vi "speis.vi"(0 "IP adress":string="192.109.209.229", 1 "stop":bool, 2 "Channel":u8(ring)=4 items=["1", "2", "3", "4", "5", "6", "7", "8", "9", "10", "11", "12", "13", "14", "15", "16"], 3 "SPEIS Parameters":T2={"Step_number"=2, "Initial_Voltage_step"=0.0, "vs_initial"=TRUE, "Final_Voltage_step"=1.0, "vs_final"=FALSE, "Duration_step"=1.0, "Record_every_dI"=0.1, "Record_every_dT"=0.1, "Initial_frequency"=100000.0, "sweep"=FALSE, "Final_frequency"=1.0, "Frequency_number"=51, "Amplitude_Voltage"=0.01, "Wait_for_steady"=2.0, "Average_N_times"=1, "Correction"=TRUE, "I_Range"=12, "Bandwidth"=5, "em"=1, "ce"=0} {"ce" items=["Standard", "CE to ground"]; "Initial_Voltage_step" min=-10 max=10 format="%.5f"; "Step_number" min=0 step=1; "I_Range" items=["1pA", "1nA", "10nA", "100nA", "1µA", "10µA", "100µA", "1mA", "10mA", "100mA", "1A", "Booster", "Auto"]; "Wait_for_steady" min=0 format="%.2f"; "Record_every_dT" min=0 format="%.2e"; "Record_every_dI" min=0 format="%.2e"; "Duration_step" min=0 format="%.5f"; "Final_Voltage_step" min=-10 max=10 format="%.5f"; "Bandwidth" items=["1"=1, "2"=2, "3"=3, "4"=4, "5"=5, "6"=6, "7"=7, "8"=8, "9"=9]; "Average_N_times" min=1 max=1000 step=1; "Amplitude_Voltage" min=0.0005 max=0.5 format="%.2e"; "Final_frequency" min=1e-05 max=1000000 format="%.2e"; "Frequency_number" min=1 max=10000; "Initial_frequency" min=1e-05 max=1000000 format="%.2e"}, 4 "Exit":bool, 5 "Start":bool, 8 "Draw":T1(ring)) -> (6 "XY Graph":cluster{"Data p1":sgl[], "Data p1":dbl[]}[](graph)=[{"Data p1"=[525.50006, 538.618, 558.7457, 587.3537, 630.11804, 690.5473, 769.1625, 866.5284, 976.17816, 1089.6279, 1189.7482, 1279.7397, 1345.3214, 1394.7092, 1431.7653, 1455.0223, 1469.8767, 1479.4921, 1485.3942, 1488.4973, 1493.599, 1495.9125, 1499.4656, 1502.3853, 1506.3972, 1509.198, 1519.7369, 1532.5125, 1548.5372, 1580.3093, 1625.0144, 1694.3768, 1801.5819, 1957.731, 2171.8762, 2461.144, 2817.8232, 3216.9392, 3619.0576, 3986.1555, 4300.8384, 4536.2026, 4707.0835, 4828.639, 4904.999, 4961.0366, 4994.4067, 5015.1143, 5029.5254, 5037.418, 5042.429, 525.3447, 538.11237, 558.4203, 587.67224, 630.1018, 689.9828, 768.2711, 865.9559, 975.45575, 1088.0951, 1190.5238, 1279.0249, 1347.1433, 1396.1802, 1430.4937, 1455.2814, 1469.1127, 1480.9547, 1488.2792, 1491.4941, 1493.8552, 1496.4435, 1497.5511, 1502.2585, 1506.1387, 1509.9863, 1518.135, 1530.0344, 1549.0596, 1579.7124, 1625.0818, 1698.2051, 1802.8951, 1952.263, 2172.5627, 2465.0474, 2821.2722, 3224.1062, 3621.5154, 4006.4937, 4287.0464, 4530.4033, 4711.4463, 4846.2896, 4918.22, 4963.792, 5006.571, 5024.125, 5036.2017, 5047.449, 5051.315, 525.54193, 538.3897, 557.91473, 588.05676, 630.4936, 689.3102, 769.6545, 866.44385, 976.8946, 1088.5287, 1191.8607, 1279.7543, 1347.9636, 1396.8135, 1430.9287, 1453.9589, 1470.3905, 1480.8995, 1486.5005, 1491.8065, 1494.8728, 1495.035, 1497.364, 1502.3115, 1506.6406, 1509.7494, 1520.2966, 1532.3849, 1551.5309, 1581.3643, 1626.9884, 1696.2556, 1800.7041, 1954.6533, 2176.5808, 2462.342, 2819.6333, 3220.7124, 3630.4177, 3998.0688, 4306.804, 4559.2373, 4719.661, 4837.343, 4913.759, 4967.9824, 5011.7876, 5025.0054, 5040.9824, 5049.399, 5058.189], "Data p1"=[-150.71189880371094, -185.61993408203125, -228.1602783203125, -277.7409362792969, -332.0828552246094, -388.3536071777344, -440.2685852050781, -479.6073303222656, -497.4354248046875, -492.5791931152344, -463.5277404785156, -416.0335998535156, -364.6885070800781, -311.1602783203125, -263.2023010253906, -222.48780822753906, -189.07347106933594, -164.32290649414062, -147.07318115234375, -137.23709106445312, -134.4752197265625, -138.10047912597656, -152.14559936523438, -170.2203369140625, -199.28997802734375, -238.3840789794922, -290.4477233886719, -355.0041809082031, -435.4027404785156, -539.1777954101562, -667.4210815429688, -821.8733520507812, -997.7675170898438, -1197.373291015625, -1394.82568359375, -1582.048095703125, -1717.46923828125, -1778.4962158203125, -1742.513427734375, -1633.1392822265625, -1453.841064453125, -1255.0560302734375, -1052.457275390625, -865.8721923828125, -707.827880859375, -570.5523681640625, -455.1785888671875, -364.49017333984375, -289.9132995605469, -231.135009765625, -183.6439971923828, -150.6773681640625, -185.84783935546875, -228.77284240722656, -278.3961181640625, -332.7877502441406, -388.551513671875, -440.7836608886719, -479.08306884765625, -499.46099853515625, -492.4226989746094, -464.9497985839844, -416.5841979980469, -364.1741027832031, -310.4356994628906, -262.843017578125, -223.28204345703125, -189.56234741210938, -164.49154663085938, -148.58004760742188, -137.69810485839844, -135.09109497070312, -138.912841796875, -151.2158966064453, -170.32308959960938, -196.95445251464844, -236.5548095703125, -289.3612976074219, -354.9062194824219, -435.35992431640625, -540.9880981445312, -668.5939331054688, -821.7505493164062, -993.9796752929688, -1198.608154296875, -1398.090087890625, -1581.3919677734375, -1721.475341796875, -1777.119140625, -1735.2742919921875, -1629.3763427734375, -1462.967529296875, -1237.9119873046875, -1051.7672119140625, -870.1654663085938, -707.5675048828125, -580.3982543945312, -455.0499572753906, -364.8717041015625, -287.6647033691406, -226.23031616210938, -186.34091186523438, -150.48431396484375, -185.98463439941406, -228.33602905273438, -277.496337890625, -332.2249450683594, -388.3759460449219, -440.437255859375, -480.6752624511719, -497.97943115234375, -490.92437744140625, -463.6277160644531, -416.9968566894531, -364.2229309082031, -311.0670471191406, -263.4906311035156, -221.8280487060547, -190.08363342285156, -165.50880432128906, -145.69888305664062, -135.96371459960938, -134.3701934814453, -139.62152099609375, -151.39317321777344, -170.60525512695312, -198.75314331054688, -237.4167022705078, -288.7137756347656, -355.7140808105469, -437.6841735839844, -539.8258666992188, -668.255859375, -819.745361328125, -995.9793701171875, -1194.9197998046875, -1398.14892578125, -1591.957763671875, -1718.02490234375, -1787.792236328125, -1749.94580078125, -1622.7584228515625, -1456.0980224609375, -1251.5211181640625, -1044.2322998046875, -868.7525024414062, -706.819580078125, -570.400390625, -455.4763488769531, -364.127197265625, -294.8734130859375, -231.19313049316406, -184.1147003173828]}], 7 "Number of points":i32=153)   [LabVIEW 2012]
doc: "The Staircase Potentio Electrochemical Impedance Spectroscopy (SPEIS) technique is designed to perform successive impedance measurements (on a whole frequency range) during a potential sweep. \nThis technique consists in a staircase potential sweep (potential limits and number of steps defined by the user). An impedance measurement (with an adjustable number of frequencies) is performed on each potential step.\n\nIn general, in this VI, the first thing to do is to start by establishing the connection with the instrument defined by its IP adress, then load the firmware in the channel selected, get the information on the plugged channels, load protocol on a channel, start/stop the protocol, retreive data and draw the graph.\nThis technique is applied just for channels with impedance capabilities (Zboard)."
uses:
  base_xml.llb/Type Descriptor Enumeration__ogtk.ctl
panel:
  out "Data p0":sgl[][](array[numeric])=[[0.100008, 0.0009844337, 1.788816e-07, 1.0], [0.200016, 0.0010607007, 1.7521837e-07, 1.0], [0.300024, 0.0009844337, 1.7453168e-07, 1.0], [0.400032, 0.0009844337, 1.7399759e-07, 1.0], [0.50004, 0.0010607007, 1.7369238e-07, 1.0], [0.600048, 0.0007556325, 1.7285309e-07, 1.0], [0.700056, 0.0010607007, 1.7415019e-07, 1.0], [0.800064, 0.0009844337, 1.732346e-07, 1.0], [0.90007204, 0.00090816664, 1.729294e-07, 1.0], [31.67708, 0.5012512, 9.935654e-05, 1.0000001], [31.777088, 0.5012512, 9.9204015e-05, 1.0000001], [31.877096, 0.50132746, 9.912774e-05, 1.0000001], [31.977104, 0.50148, 9.935654e-05, 1.0000001], [32.07711, 0.5012512, 9.9204015e-05, 1.0000001], [32.17712, 0.5012512, 9.9204015e-05, 1.0000001], [32.277126, 0.5012512, 9.912774e-05, 1.0000001], [32.377136, 0.50132746, 9.9204015e-05, 1.0000001], [32.477142, 0.5011749, 9.912774e-05, 1.0000001], [60.111145, 0.96091276, 0.000400375, 1.0000002], [60.21115, 1.0013343, 0.00019804362, 1.0000002], [60.31116, 1.001258, 0.00019819614, 1.0000002], [60.411167, 1.0013343, 0.0001982724, 1.0000002], [60.511177, 1.0013343, 0.00019819614, 1.0000002], [60.611183, 1.0015631, 0.00019811987, 1.0000002], [60.711193, 1.001258, 0.00019819614, 1.0000002], [60.8112, 1.0013343, 0.0001982724, 1.0000002], [60.91121, 1.001258, 0.00019796735, 1.0000002], [61.011215, 1.001258, 0.00019804362, 1.0000002]]
  out "Data p1":sgl[][](array[numeric])=[[100031.24, 0.009869354, 1.8053093e-05, -0.27930045, 0.001764305, 3.9379972e-07, 0.0, 0.018222777, 1.8088715e-05, -0.025958419, -0.00018480215, -3.9379972e-07, 2.0, 2.029, 8.0, 1.0], [79437.5, 0.010228618, 1.7954228e-05, -0.33187628, 0.0017653664, 3.8618438e-07, 0.0, 0.01806867, 1.7994063e-05, -0.018080682, -0.00019200613, -3.861844e-07, 2.0, 2.114, 8.0, 1.0], [63093.75, 0.010669165, 1.7677803e-05, -0.3876784, 0.0017698539, 3.946376e-07, 0.0, 0.017742673, 1.7717768e-05, -0.015037537, -0.00018748268, -3.946376e-07, 2.0, 2.199, 8.0, 1.0], [50125.0, 0.0101253055, 1.5584323e-05, -0.44170764, 0.0017671726, 3.9245887e-07, 0.0, 0.015633836, 1.5619022e-05, -0.011037588, -0.00018580719, -3.924589e-07, 2.0, 2.368, 8.0, 1.0], [39812.496, 0.010687894, 1.5005408e-05, -0.48502678, 0.0017727586, 3.9467452e-07, 0.0, 0.015032693, 1.5036869e-05, -0.009105086, -0.00020297953, -3.9467454e-07, 2.0, 2.453, 8.0, 1.0], [31625.002, 0.010131325, 1.27878975e-05, -0.5123023, 0.0017680849, 3.9675982e-07, 0.0, 0.012788134, 1.2812633e-05, -0.005294323, -0.00019100076, -3.9675984e-07, 2.0, 2.622, 8.0, 1.0], [25124.996, 0.010685012, 1.2056367e-05, -0.51987815, 0.0017704311, 3.8622122e-07, 0.0, 0.012053828, 1.2077107e-05, -0.0034683943, -0.00018999552, -3.8622125e-07, 2.0, 2.707, 8.0, 1.0], [19953.123, 0.010150351, 1.0248726e-05, -0.5055121, 0.001768178, 3.9500952e-07, 0.0, 0.010238029, 1.0263841e-05, -0.0036523342, -0.00019217345, -3.9500955e-07, 2.0, 2.876, 8.0, 1.0], [15842.013, 0.010598964, 9.674011e-06, -0.4712778, 0.0017736709, 3.9139732e-07, 0.0, 0.009650077, 9.6858e-06, -0.0015640259, -0.00019803717, -3.9139735e-07, 2.0, 2.961, 8.0, 1.0], [12590.899, 0.010097275, 8.443992e-06, -0.42456722, 0.0017629458, 3.7616655e-07, 0.0, 0.008435441, 8.452159e-06, 2.670288e-05, -0.00016000666, -3.7616658e-07, 2.0, 3.161, 8.0, 1.0], [10019.525, 0.0104980795, 8.221826e-06, -0.3715102, 0.0017539338, 3.6335635e-07, 0.0, 0.008224506, 8.227834e-06, -0.00051116943, -0.0001420804, -3.633564e-07, 2.0, 3.28, 8.0, 1.0], [7944.256, 0.010987763, 8.165296e-06, -0.31431544, 0.0017541572, 3.568768e-07, 0.0, 0.0081453305, 8.16958e-06, -0.0020017624, -0.00012088722, -3.5687682e-07, 2.0, 3.425, 8.0, 1.0], [6322.935, 0.010157951, 7.287563e-06, -0.26471734, 0.0017405088, 3.52557e-07, 0.0, 0.0072648395, 7.2902762e-06, 0.0013228655, -0.00012222746, -3.5255704e-07, 2.0, 3.778, 8.0, 1.0], [5013.0186, 0.01075666, 7.5274156e-06, -0.21950568, 0.0017390565, 3.5142125e-07, 0.0, 0.00750066, 7.529323e-06, -0.0017416477, -0.0001242379, -3.5142128e-07, 2.0, 3.992, 8.0, 1.0], [3981.1804, 0.010172644, 6.987874e-06, -0.18180084, 0.0017367104, 3.4957787e-07, 0.0, 0.0069908933, 6.9890734e-06, -0.0010359287, -0.00012180861, -3.4957793e-07, 2.0, 4.42, 8.0, 1.0], [3160.0593, 0.010855657, 7.3750953e-06, -0.15173492, 0.0017394476, 3.489076e-07, 0.0, 0.007377897, 7.375971e-06, -0.00044322014, -0.00012591323, -3.4890766e-07, 2.0, 4.6349998, 8.0, 1.0], [2514.0195, 0.010156401, 6.853231e-06, -0.12792969, 0.0017408812, 3.498758e-07, 0.0, 0.006835944, 6.8537975e-06, 0.0020416975, -0.00014182905, -3.4987585e-07, 2.0, 5.062, 8.0, 1.0], [1993.0898, 0.010699353, 7.1875784e-06, -0.11061376, 0.001741235, 3.443086e-07, 0.0, 0.007164294, 7.1879995e-06, -0.0009522438, -0.00013546273, -3.4430863e-07, 2.0, 5.277, 8.0, 1.0], [1583.4792, 0.010107939, 6.771774e-06, -0.098691225, 0.0017376042, 3.4693392e-07, 0.0, 0.006733144, 6.7720653e-06, -0.0009715855, -0.00013630038, -3.4693397e-07, 2.0, 5.708, 8.0, 1.0], [1258.7904, 0.010411834, 6.965321e-06, -0.091938496, 0.001736487, 3.3749387e-07, 0.0, 0.0069400347, 6.965549e-06, -0.0020059347, -0.00013872965, -3.3749393e-07, 2.0, 5.9240003, 8.0, 1.0], [999.0409, 0.010659541, 7.108064e-06, -0.08979225, 0.0017378834, 3.385552e-07, 0.0, 0.0071048443, 7.108256e-06, -3.9339066e-06, -0.00013093927, -3.3855522e-07, 2.0, 6.1410003, 8.0, 1.0], [794.2393, 0.010820501, 7.2027497e-06, -0.092057616, 0.0017324092, 3.4103158e-07, 0.0, 0.007164113, 7.2029206e-06, 0.0011003017, -0.000125997, -3.4103164e-07, 2.0, 6.3580003, 8.0, 1.0], [631.00977, 0.010931326, 7.2529074e-06, -0.10112047, 0.0017288156, 3.4155292e-07, 0.0, 0.0072435015, 7.2530606e-06, 0.0020492077, -0.0001239028, -3.4155298e-07, 2.0, 6.576, 8.0, 1.0], [500.80118, 0.010105555, 6.683579e-06, -0.11281896, 0.001734774, 3.4153427e-07, 0.0, 0.006647158, 6.683726e-06, -0.0010091066, -0.00013177695, -3.4153433e-07, 2.0, 7.0090003, 8.0, 1.0], [398.5971, 0.010142034, 6.674487e-06, -0.13153195, 0.0017367849, 3.433962e-07, 0.0, 0.006641871, 6.6746197e-06, 0.0012131929, -0.00015238376, -3.4339627e-07, 2.0, 7.229, 8.0, 1.0], [316.3159, 0.0101667335, 6.654018e-06, -0.15665984, 0.0017379579, 3.4335898e-07, 0.0, 0.0066457815, 6.654146e-06, -0.001480341, -0.00015380779, -3.4335903e-07, 2.0, 7.448, 8.0, 1.0], [251.04433, 0.01018918, 6.585379e-06, -0.18883991, 0.0017377159, 3.436569e-07, 0.0, 0.0065762023, 6.5854924e-06, 0.002457559, -0.00014300179, -3.4365695e-07, 2.0, 7.669, 8.0, 1.0], [199.29855, 0.010201627, 6.4850747e-06, -0.22763349, 0.001744326, 3.450161e-07, 0.0, 0.0064792074, 6.485203e-06, -0.0012426376, -0.00014953566, -3.4501616e-07, 2.0, 7.895, 8.0, 1.0], [158.62956, 0.01019249, 6.3363113e-06, -0.27409363, 0.0017508802, 3.4900066e-07, 0.0, 0.0063282293, 6.336429e-06, -0.00015228987, -0.00014551482, -3.4900071e-07, 2.0, 8.123, 8.0, 1.0], [125.84552, 0.010199593, 6.108428e-06, -0.32880032, 0.0017499119, 3.396537e-07, 0.0, 0.006088465, 6.10855e-06, -0.0021110773, -0.00014844669, -3.3965375e-07, 2.0, 8.351, 8.0, 1.0], [99.90408, 0.010190543, 5.8008377e-06, -0.3897109, 0.0017508056, 3.446437e-07, 0.0, 0.005801017, 5.8009496e-06, 0.0016998751, -0.00014727394, -3.4464375e-07, 2.0, 8.585, 8.0, 1.0], [79.51632, 0.010190832, 5.4114853e-06, -0.4516238, 0.0017413839, 3.3969093e-07, 0.0, 0.005403216, 5.4116135e-06, -0.0005774498, -0.00014107513, -3.3969098e-07, 2.0, 8.826, 8.0, 1.0], [63.160732, 0.0101588145, 4.932837e-06, -0.50577784, 0.0017380696, 3.232843e-07, 0.0, 0.0048995684, 4.933435e-06, -0.0022892952, -0.00015162982, -3.2328435e-07, 2.0, 9.331, 7.0, 1.0], [50.08012, 0.0101338, 4.4158555e-06, -0.5489146, 0.0017423521, 3.2462907e-07, 0.0, 0.0044069523, 4.416364e-06, -0.0016965866, -0.00016863461, -3.2462918e-07, 2.0, 9.584, 7.0, 1.0], [39.85971, 0.010110853, 3.917116e-06, -0.57088757, 0.0017390565, 3.232749e-07, 0.0, 0.003909233, 3.917622e-06, 0.0017719865, -0.0001569909, -3.23275e-07, 2.0, 9.849, 7.0, 1.0], [31.58696, 0.010090547, 3.4488567e-06, -0.5713042, 0.001736487, 3.2309606e-07, 0.0, 0.0034521155, 3.4493996e-06, -0.003828764, -0.00017081253, -3.2309612e-07, 2.0, 10.116, 7.0, 1.0], [25.104433, 0.010081783, 3.05511e-06, -0.5473771, 0.0017249426, 3.2149413e-07, 0.0, 0.0030513897, 3.0555955e-06, 0.0057106614, -0.00014534722, -3.2149427e-07, 2.0, 10.409, 7.0, 1.0], [19.929855, 0.010076249, 2.7412152e-06, -0.5050314, 0.0017313849, 3.2125197e-07, 0.0, 0.0027353163, 2.7417095e-06, -0.0069835186, -0.00015146224, -3.212521e-07, 2.0, 10.725, 7.0, 1.0], [15.836134, 0.010059833, 2.5044978e-06, -0.44872427, 0.0017287785, 3.204436e-07, 0.0, 0.0025177128, 2.5049212e-06, 0.009344101, -0.00014677126, -3.2044363e-07, 2.0, 11.055, 7.0, 1.0], [12.600794, 0.010063741, 2.3362027e-06, -0.38884282, 0.0017246262, 3.186163e-07, 0.0, 0.0023388118, 2.3364873e-06, 0.0006400645, -0.00014635241, -3.186164e-07, 2.0, 11.465, 7.0, 1.0], [9.990409, 0.010058779, 2.2156298e-06, -0.32597756, 0.0017271581, 3.216877e-07, 0.0, 0.0022162707, 2.2159718e-06, -0.0044992566, -0.00015028955, -3.21688e-07, 2.0, 11.879, 7.0, 1.0], [7.939562, 0.010051124, 2.1355277e-06, -0.2699232, 0.0017190769, 3.1830135e-07, 0.0, 0.0021537226, 2.1358414e-06, -0.0010365248, -0.00014350438, -3.1830172e-07, 2.0, 12.397, 7.0, 1.0], [6.3004045, 0.010050946, 2.0838283e-06, -0.21997207, 0.0017442836, 3.3078075e-07, 0.0, 0.0020929575, 2.084185e-06, 0.00019574165, -0.00018570227, -3.307811e-07, 2.0, 13.045, 7.0, 1.0], [5.008012, 0.010055232, 2.049721e-06, -0.17743433, 0.001757515, 3.327263e-07, 0.0, 0.002057552, 2.0499922e-06, -0.0017228127, -0.00021201238, -3.3272647e-07, 2.0, 13.857, 7.0, 1.0], [3.9859712, 0.010047529, 2.027425e-06, -0.14331807, 0.0017548279, 3.3264936e-07, 0.0, 0.0020328981, 2.0277243e-06, -0.0021646023, -0.00020486997, -3.326495e-07, 2.0, 14.873, 7.0, 1.0], [3.1680837, 0.010054357, 2.0133932e-06, -0.11450362, 0.0017575176, 3.332066e-07, 0.0, 0.0020133706, 2.0137181e-06, 0.0010950565, -0.00020909487, -3.3320666e-07, 2.0, 16.148, 7.0, 1.0], [2.504006, 0.010050174, 2.0039806e-06, -0.09088659, 0.0017548916, 3.3225882e-07, 0.0, 0.002016635, 2.0043522e-06, -0.00028324127, -0.00023046214, -3.3225888e-07, 2.0, 17.759, 7.0, 1.0], [1.9879117, 0.010061348, 2.0009275e-06, -0.07255077, 0.0017483011, 3.1155264e-07, 0.0, 0.0020140824, 2.0043926e-06, -0.003084302, -0.00021901223, -3.1155272e-07, 2.0, 21.81, 6.0, 1.0], [1.5814751, 0.010062281, 1.9973268e-06, -0.057578564, 0.0017498633, 3.115516e-07, 0.0, 0.002005952, 2.0001908e-06, -0.0011792183, -0.00022941067, -3.1155167e-07, 2.0, 24.351, 6.0, 1.0], [1.2617111, 0.010061398, 1.9952333e-06, -0.04585147, 0.0017614333, 3.124857e-07, 0.0, 0.002001588, 1.9988286e-06, -0.00019466877, -0.00024342869, -3.124858e-07, 2.0, 27.535, 6.0, 1.0], [1.0000616, 0.010060886, 1.993924e-06, -0.036403656, 0.0017541798, 3.1092628e-07, 0.0, 0.0020091715, 1.9974327e-06, 0.0009430647, -0.00025171688, -3.109264e-07, 2.0, 31.547, 6.0, 1.0], [100031.24, 0.0098445695, 1.8012992e-05, -0.2793181, 0.5023526, 9.9444e-05, 0.0, 0.018171087, 1.8048326e-05, -0.026801586, -0.09870481, -9.9444056e-05, 2.0, 32.842, 8.0, 1.0000001], [79437.5, 0.010201275, 1.7918928e-05, -0.3325441, 0.5023489, 9.944558e-05, 0.0, 0.018042367, 1.7958415e-05, -0.019655943, -0.09869501, -9.944564e-05, 2.0, 32.927, 8.0, 1.0000001], [63093.75, 0.0106439395, 1.7638034e-05, -0.38882208, 0.50235265, 9.943754e-05, 0.0, 0.017762726, 1.767797e-05, -0.015104622, -0.09869928, -9.9437595e-05, 2.0, 33.012, 8.0, 1.0000001], [50125.0, 0.0101334, 1.5583151e-05, -0.44240904, 0.5023567, 9.944524e-05, 0.0, 0.015648432, 1.561785e-05, -0.01154542, -0.09869794, -9.944531e-05, 2.0, 33.181, 8.0, 1.0000001], [39812.496, 0.010694962, 1.50087035e-05, -0.48591256, 0.50235, 9.944413e-05, 0.0, 0.01505019, 1.5040246e-05, -0.0089610815, -0.09870121, -9.944419e-05, 2.0, 33.266, 8.0, 1.0000001], [31625.002, 0.010122286, 1.278286e-05, -0.5128696, 0.50235736, 9.944271e-05, 0.0, 0.012805648, 1.2807578e-05, -0.00564456, -0.09869266, -9.9442776e-05, 2.0, 33.435, 8.0, 1.0000001], [25124.996, 0.01068203, 1.2060042e-05, -0.5208827, 0.50235415, 9.944534e-05, 0.0, 0.01207983, 1.2080859e-05, -0.002794981, -0.0986992, -9.9445395e-05, 2.0, 33.52, 8.0, 1.0000001], [19953.123, 0.010127757, 1.0233712e-05, -0.5053288, 0.50235045, 9.9442674e-05, 0.0, 0.0102022225, 1.02488275e-05, -0.0020895004, -0.09868982, -9.944273e-05, 2.0, 33.689, 8.0, 1.0000001], [15842.013, 0.010588318, 9.661842e-06, -0.47322392, 0.5023422, 9.944442e-05, 0.0, 0.009648947, 9.67358e-06, -0.0046185255, -0.09871059, -9.9444485e-05, 2.0, 33.774, 8.0, 1.0000001], [12590.899, 0.010092828, 8.450599e-06, -0.4249765, 0.50233316, 9.9429526e-05, 0.0, 0.00844272, 8.45875e-06, -0.0016593933, -0.09873647, -9.942959e-05, 2.0, 33.974, 8.0, 1.0000001], [10019.525, 0.010512863, 8.22542e-06, -0.3723266, 0.50232905, 9.941938e-05, 0.0, 0.008206242, 8.231428e-06, -0.0018035471, -0.09876336, -9.941944e-05, 2.0, 34.093, 8.0, 1.0000001], [7944.256, 0.010984279, 8.165798e-06, -0.314869, 0.50230646, 9.942549e-05, 0.0, 0.008157445, 8.170098e-06, -0.0006506443, -0.09879143, -9.942555e-05, 2.0, 34.238, 8.0, 1.0000001], [6322.935, 0.010159299, 7.2800467e-06, -0.26401997, 0.50230694, 9.942065e-05, 0.0, 0.0072693247, 7.2827347e-06, -0.000656724, -0.098796874, -9.942071e-05, 2.0, 34.591, 8.0, 1.0000001], [5013.0186, 0.01076707, 7.5279663e-06, -0.21878731, 0.5023011, 9.9421966e-05, 0.0, 0.0075109596, 7.5298844e-06, 0.0021368265, -0.098802485, -9.942203e-05, 2.0, 34.805, 8.0, 1.0000001], [3981.1804, 0.010141009, 6.972445e-06, -0.18171597, 0.5023099, 9.94204e-05, 0.0, 0.0069551812, 6.973644e-06, -0.0014134645, -0.098800726, -9.942047e-05, 2.0, 35.232998, 8.0, 1.0000001], [3160.0593, 0.010814573, 7.345306e-06, -0.15224159, 0.5023008, 9.941756e-05, 0.0, 0.00732549, 7.34618e-06, 0.00026023388, -0.09881589, -9.9417615e-05, 2.0, 35.447998, 8.0, 1.0000001], [2514.0195, 0.010146751, 6.849933e-06, -0.12832284, 0.5023021, 9.9421355e-05, 0.0, 0.006846147, 6.8504905e-06, -0.00093489885, -0.09882795, -9.942141e-05, 2.0, 35.875, 8.0, 1.0000001], [1993.0898, 0.010708808, 7.1868208e-06, -0.110617876, 0.5023014, 9.942003e-05, 0.0, 0.007165335, 7.187241e-06, 9.0539455e-05, -0.09881589, -9.94201e-05, 2.0, 36.09, 8.0, 1.0000001], [1583.4792, 0.010109009, 6.7588167e-06, -0.099503756, 0.502314, 9.942188e-05, 0.0, 0.0067454996, 6.7591172e-06, -0.0013484955, -0.09880408, -9.942194e-05, 2.0, 36.521, 8.0, 1.0000001], [1258.7904, 0.01042904, 6.962733e-06, -0.09206128, 0.50230646, 9.9420424e-05, 0.0, 0.006942235, 6.9629655e-06, -0.0010188818, -0.09880961, -9.942048e-05, 2.0, 36.737, 8.0, 1.0000001], [999.0409, 0.010662441, 7.108527e-06, -0.09018588, 0.502309, 9.942275e-05, 0.0, 0.0071001127, 7.108718e-06, 0.0004374683, -0.09881723, -9.942281e-05, 2.0, 36.954, 8.0, 1.0000001], [794.2393, 0.010825973, 7.203498e-06, -0.09256339, 0.502312, 9.941892e-05, 0.0, 0.00717161, 7.203662e-06, 0.00017946959, -0.098821, -9.9418976e-05, 2.0, 37.171, 8.0, 1.0000001], [631.00977, 0.010925124, 7.258416e-06, -0.10063434, 0.50231636, 9.9420366e-05, 0.0, 0.007239861, 7.258568e-06, 0.000377357, -0.09881304, -9.942043e-05, 2.0, 37.389, 8.0, 1.0000001], [500.80118, 0.010092256, 6.675288e-06, -0.11289591, 0.50231606, 9.942469e-05, 0.0, 0.0066652843, 6.675438e-06, 0.002040863, -0.098825686, -9.9424746e-05, 2.0, 37.822, 8.0, 1.0000001], [398.5971, 0.010133827, 6.671549e-06, -0.13002998, 0.5023148, 9.9419434e-05, 0.0, 0.0066457107, 6.6716825e-06, -0.0009510517, -0.09882535, -9.94195e-05, 2.0, 38.042, 8.0, 1.0000001], [316.3159, 0.010161628, 6.6485254e-06, -0.15539718, 0.502312, 9.9416065e-05, 0.0, 0.006621068, 6.6486464e-06, -0.00054088235, -0.098803654, -9.9416124e-05, 2.0, 38.261, 8.0, 1.0000001], [251.04433, 0.010178372, 6.5859585e-06, -0.188344, 0.5023104, 9.941789e-05, 0.0, 0.006556802, 6.5860772e-06, -0.005339384, -0.09880474, -9.941795e-05, 2.0, 38.482, 8.0, 1.0000001], [199.29855, 0.010187284, 6.4860014e-06, -0.22792876, 0.5023066, 9.941765e-05, 0.0, 0.0064526796, 6.486125e-06, -0.0012413263, -0.09880517, -9.941771e-05, 2.0, 38.708, 8.0, 1.0000001], [158.62956, 0.0101962155, 6.336692e-06, -0.27398014, 0.5023068, 9.942128e-05, 0.0, 0.006298506, 6.336816e-06, -0.0003578663, -0.0987993, -9.942134e-05, 2.0, 38.936, 8.0, 1.0000001], [125.84552, 0.010186324, 6.1004052e-06, -0.3299418, 0.502307, 9.942126e-05, 0.0, 0.006089459, 6.100529e-06, 0.001291275, -0.09882083, -9.9421326e-05, 2.0, 39.164, 8.0, 1.0000001], [99.90408, 0.010190524, 5.799149e-06, -0.39031374, 0.502313, 9.942007e-05, 0.0, 0.005785656, 5.7992693e-06, 0.0025515556, -0.09880784, -9.942013e-05, 2.0, 39.398, 8.0, 1.0000001], [79.51632, 0.010190615, 5.4016414e-06, -0.45067966, 0.5023128, 9.942009e-05, 0.0, 0.0054049282, 5.4017673e-06, 0.0016866922, -0.098816976, -9.942015e-05, 2.0, 39.639, 8.0, 1.0000001], [63.160732, 0.010182999, 4.946219e-06, -0.5038593, 0.5023102, 9.941584e-05, 0.0, 0.004933287, 4.9463183e-06, 0.0018147826, -0.0988261, -9.9415905e-05, 2.0, 39.891, 8.0, 1.0000001], [50.08012, 0.010176448, 4.442216e-06, -0.5506198, 0.50231785, 9.941849e-05, 0.0, 0.004437907, 4.4423036e-06, -0.0029598475, -0.09882468, -9.941855e-05, 2.0, 40.144, 8.0, 1.0000001], [39.85971, 0.010174631, 3.9382503e-06, -0.5718072, 0.50231034, 9.94172e-05, 0.0, 0.0039190855, 3.9383317e-06, 0.002768755, -0.09881706, -9.941726e-05, 2.0, 40.409, 8.0, 1.0000001], [31.58696, 0.0101682935, 3.4719528e-06, -0.570395, 0.50230974, 9.941443e-05, 0.0, 0.0034850314, 3.4720297e-06, -0.0012363754, -0.09881279, -9.941449e-05, 2.0, 40.676, 8.0, 1.0000001], [25.104433, 0.010180413, 3.0803023e-06, -0.54786897, 0.50230956, 9.94161e-05, 0.0, 0.0030881276, 3.0803697e-06, -0.0059039593, -0.09880047, -9.941617e-05, 2.0, 40.969, 8.0, 1.0000001], [19.929855, 0.010168958, 2.7622218e-06, -0.5037621, 0.50231475, 9.941813e-05, 0.0, 0.0027613966, 2.7622877e-06, 0.0041599274, -0.09882351, -9.94182e-05, 2.0, 41.285, 8.0, 1.0000001], [15.836134, 0.010177033, 2.5342558e-06, -0.44683456, 0.50230587, 9.941377e-05, 0.0, 0.002547863, 2.534308e-06, 8.249283e-05, -0.09882167, -9.941384e-05, 2.0, 41.615, 8.0, 1.0000001], [12.600794, 0.010165244, 2.350268e-06, -0.38625503, 0.5023023, 9.940979e-05, 0.0, 0.0023703233, 2.3503023e-06, 0.0055634975, -0.09882477, -9.940985e-05, 2.0, 42.025, 8.0, 1.0000001], [9.990409, 0.010168751, 2.244859e-06, -0.32886124, 0.50231725, 9.941567e-05, 0.0, 0.0022310652, 2.2448912e-06, -0.0013589859, -0.09881782, -9.941574e-05, 2.0, 42.439, 8.0, 1.0000001], [7.939562, 0.010161909, 2.163726e-06, -0.26673427, 0.50229883, 9.94073e-05, 0.0, 0.002151734, 2.163761e-06, 0.0018897057, -0.09882644, -9.9407356e-05, 2.0, 42.957, 8.0, 1.0000001], [6.3004045, 0.010165019, 2.1056856e-06, -0.21963537, 0.50234437, 9.944084e-05, 0.0, 0.0021051469, 2.105732e-06, 0.0015662909, -0.0987485, -9.94409e-05, 2.0, 43.605, 8.0, 1.0000001], [5.008012, 0.010162866, 2.0640332e-06, -0.17765987, 0.50236815, 9.944183e-05, 0.0, 0.0020733313, 2.0640725e-06, 0.0015951991, -0.09871536, -9.9441895e-05, 2.0, 44.417, 8.0, 1.0000001], [3.9859712, 0.010170557, 2.0468603e-06, -0.14288616, 0.5023549, 9.944426e-05, 0.0, 0.002051187, 2.046899e-06, -0.0023578405, -0.09872899, -9.944432e-05, 2.0, 45.433, 8.0, 1.0000001], [3.1680837, 0.010164456, 2.0338641e-06, -0.11639786, 0.50236046, 9.944176e-05, 0.0, 0.0020320597, 2.0339014e-06, -0.0016188174, -0.098730944, -9.944182e-05, 2.0, 46.708, 8.0, 1.0000001], [2.504006, 0.010165603, 2.022117e-06, -0.0906415, 0.50235975, 9.943858e-05, 0.0, 0.0020237681, 2.0221569e-06, 0.001527816, -0.09872592, -9.9438636e-05, 2.0, 48.319, 8.0, 1.0000001], [1.9879117, 0.010163971, 2.017719e-06, -0.07249665, 0.50236595, 9.9442696e-05, 0.0, 0.00201306, 2.017754e-06, 0.0034449697, -0.09872519, -9.944276e-05, 2.0, 50.344, 8.0, 1.0000001], [1.5814751, 0.010166594, 2.0154175e-06, -0.05705738, 0.5023677, 9.943813e-05, 0.0, 0.0020167315, 2.0154453e-06, 0.0026154518, -0.098741725, -9.943819e-05, 2.0, 52.885002, 8.0, 1.0000001], [1.2617111, 0.010165211, 2.0119105e-06, -0.044790745, 0.50237393, 9.9441204e-05, 0.0, 0.0020097687, 2.0119444e-06, -0.0011878014, -0.098741435, -9.944127e-05, 2.0, 56.069, 8.0, 1.0000001], [1.0000616, 0.010165339, 2.0110465e-06, -0.036872864, 0.50236887, 9.943485e-05, 0.0, 0.0020112505, 2.011079e-06, -0.00036787987, -0.098736465, -9.943492e-05, 2.0, 60.081, 8.0, 1.0000001], [100031.24, 0.009874203, 1.8062705e-05, -0.27887917, 1.0023965, 0.00019837101, 0.0, 0.018217867, 1.8098304e-05, -0.025908828, -0.1974324, -0.00019837113, 2.0, 61.376, 8.0, 1.0000002], [79437.5, 0.010229639, 1.7959073e-05, -0.33261216, 1.0023942, 0.00019837615, 0.0, 0.018061075, 1.7998507e-05, -0.020430863, -0.19743323, -0.00019837626, 2.0, 61.461002, 8.0, 1.0000002], [63093.75, 0.010657836, 1.7679617e-05, -0.38846946, 1.0023932, 0.00019838069, 0.0, 0.017751286, 1.7719789e-05, -0.014036059, -0.19743566, -0.00019838082, 2.0, 61.546, 8.0, 1.0000002], [50125.0, 0.010134653, 1.5585965e-05, -0.44090533, 1.0023867, 0.00019836944, 0.0, 0.015643781, 1.5620673e-05, -0.010640502, -0.19742937, -0.00019836957, 2.0, 61.715, 8.0, 1.0000002], [39812.496, 0.010695237, 1.5007321e-05, -0.48495746, 1.0023899, 0.0001983781, 0.0, 0.01505239, 1.5038939e-05, -0.0075047016, -0.19743751, -0.00019837823, 2.0, 61.8, 8.0, 1.0000002], [31625.002, 0.010126317, 1.2798815e-05, -0.51309335, 1.0023857, 0.00019837555, 0.0, 0.012833679, 1.2823481e-05, -0.0066304207, -0.1974324, -0.00019837567, 2.0, 61.969, 8.0, 1.0000002], [25124.996, 0.010713678, 1.20817485e-05, -0.5197675, 1.0023886, 0.00019837463, 0.0, 0.012117932, 1.2102506e-05, -0.0039646626, -0.1974308, -0.00019837476, 2.0, 62.054, 8.0, 1.0000002], [19953.123, 0.0101315575, 1.022517e-05, -0.5064964, 1.0023813, 0.00019837238, 0.0, 0.010250155, 1.0240328e-05, -0.0019811392, -0.19742778, -0.00019837251, 2.0, 62.223, 8.0, 1.0000002], [15842.013, 0.010588291, 9.656466e-06, -0.47142315, 1.0023811, 0.00019837155, 0.0, 0.009667257, 9.6682425e-06, -0.001144588, -0.1974288, -0.00019837166, 2.0, 62.308002, 8.0, 1.0000002], [12590.899, 0.010107332, 8.464313e-06, -0.42368364, 1.0023705, 0.00019837197, 0.0, 0.008470851, 8.472447e-06, -0.0011277199, -0.19741866, -0.0001983721, 2.0, 62.508, 8.0, 1.0000002], [10019.525, 0.010536263, 8.238794e-06, -0.37098336, 1.0023577, 0.00019836017, 0.0, 0.00823417, 8.2448305e-06, 3.33786e-05, -0.1974231, -0.0001983603, 2.0, 62.627003, 8.0, 1.0000002], [7944.256, 0.010085632, 7.4931613e-06, -0.31499267, 1.002355, 0.00019836045, 0.0, 0.0074696494, 7.497103e-06, -0.00084959343, -0.19740793, -0.00019836058, 2.0, 62.915, 8.0, 1.0000002], [6322.935, 0.010603781, 7.594179e-06, -0.2639004, 1.0023496, 0.0001983587, 0.0, 0.007583759, 7.596981e-06, -0.00197196, -0.19740157, -0.00019835882, 2.0, 63.093002, 8.0, 1.0000002], [5013.0186, 0.010130422, 7.079106e-06, -0.21912193, 1.0023454, 0.00019835478, 0.0, 0.00706417, 7.0809e-06, 0.00029429793, -0.19739051, -0.00019835492, 2.0, 63.52, 8.0, 1.0000002], [3981.1804, 0.010777407, 7.407224e-06, -0.1820997, 1.0023527, 0.00019835576, 0.0, 0.007411968, 7.4085137e-06, 0.0006392002, -0.19739017, -0.00019835588, 2.0, 63.734, 8.0, 1.0000002], [3160.0593, 0.010149703, 6.900882e-06, -0.1514008, 1.0023472, 0.00019835084, 0.0, 0.006872337, 6.9017046e-06, 0.0008326769, -0.19739453, -0.00019835096, 2.0, 64.162, 8.0, 1.0000002], [2514.0195, 0.010791578, 7.2786916e-06, -0.12856126, 1.0023531, 0.00019835614, 0.0, 0.0072643855, 7.2792905e-06, 0.00081020594, -0.19739898, -0.00019835627, 2.0, 64.376, 8.0, 1.0000002], [1993.0898, 0.010128441, 6.797066e-06, -0.11130047, 1.0023519, 0.00019835617, 0.0, 0.006788851, 6.797471e-06, 0.00013244152, -0.19739135, -0.0001983563, 2.0, 64.806, 8.0, 1.0000002], [1583.4792, 0.010558837, 7.0692754e-06, -0.09770262, 1.0023595, 0.00019835743, 0.0, 0.0070456415, 7.069585e-06, -2.1457672e-06, -0.19740786, -0.00019835755, 2.0, 65.021996, 8.0, 1.0000002], [1258.7904, 0.010896251, 7.273916e-06, -0.090889215, 1.0023547, 0.00019835359, 0.0, 0.007247542, 7.274153e-06, -0.0014419854, -0.19739193, -0.00019835372, 2.0, 65.238, 8.0, 1.0000002], [999.0409, 0.010101824, 6.7305123e-06, -0.08964646, 1.0023379, 0.00019834786, 0.0, 0.0067235464, 6.7306933e-06, -0.0012159348, -0.19739981, -0.00019834799, 2.0, 65.671, 8.0, 1.0000002], [794.2393, 0.010250201, 6.8264567e-06, -0.09312004, 1.0023456, 0.00019835378, 0.0, 0.006796502, 6.8266136e-06, -0.0017340183, -0.19740987, -0.00019835391, 2.0, 65.888, 8.0, 1.0000002], [631.00977, 0.010365989, 6.8877093e-06, -0.100764036, 1.0023531, 0.00019835851, 0.0, 0.0068579777, 6.887857e-06, 0.0027445555, -0.19740467, -0.00019835864, 2.0, 66.106, 8.0, 1.0000002], [500.80118, 0.010440068, 6.9049547e-06, -0.1130774, 1.002347, 0.00019835678, 0.0, 0.0068895486, 6.905102e-06, -0.002287984, -0.19740726, -0.00019835691, 2.0, 66.323, 8.0, 1.0000002], [398.5971, 0.010491937, 6.9039816e-06, -0.13116074, 1.0023513, 0.00019835345, 0.0, 0.0068867994, 6.904112e-06, -0.0012151599, -0.19740182, -0.00019835358, 2.0, 66.543, 8.0, 1.0000002], [316.3159, 0.010508817, 6.876134e-06, -0.15597832, 1.0023483, 0.00019835189, 0.0, 0.0068489234, 6.8762693e-06, -0.0027065277, -0.19740526, -0.000198352, 2.0, 66.762, 8.0, 1.0000002], [251.04433, 0.010532404, 6.8062177e-06, -0.18767142, 1.0023503, 0.00019835003, 0.0, 0.0067929532, 6.806337e-06, -0.0006223917, -0.19740853, -0.00019835014, 2.0, 66.983, 8.0, 1.0000002], [199.29855, 0.010541316, 6.700858e-06, -0.22809142, 1.0023519, 0.00019835193, 0.0, 0.0067024855, 6.7009923e-06, 0.0011701584, -0.19740786, -0.00019835206, 2.0, 67.209, 8.0, 1.0000002], [158.62956, 0.010552034, 6.5455847e-06, -0.27495337, 1.0023462, 0.00019834854, 0.0, 0.0065333913, 6.5457016e-06, 0.0005195737, -0.19741464, -0.00019834867, 2.0, 67.437, 8.0, 1.0000002], [125.84552, 0.010545619, 6.3110942e-06, -0.32896352, 1.0023402, 0.00019835027, 0.0, 0.0063074618, 6.3112184e-06, 0.0020734072, -0.19742393, -0.0001983504, 2.0, 67.665, 8.0, 1.0000002], [99.90408, 0.010543439, 5.9944064e-06, -0.38972354, 1.0023437, 0.00019834832, 0.0, 0.005972035, 5.9945282e-06, 0.0042753816, -0.19740106, -0.00019834845, 2.0, 67.899, 8.0, 1.0000002], [79.51632, 0.010532324, 5.5905557e-06, -0.4501723, 1.0023446, 0.00019835166, 0.0, 0.005582896, 5.590688e-06, -0.0010163784, -0.19740409, -0.00019835179, 2.0, 68.14, 8.0, 1.0000002], [63.160732, 0.010519831, 5.1121924e-06, -0.50522435, 1.0023497, 0.00019835067, 0.0, 0.005110563, 5.1122975e-06, 0.00089907646, -0.19741505, -0.0001983508, 2.0, 68.392, 8.0, 1.0000002], [50.08012, 0.010526459, 4.594778e-06, -0.5487019, 1.0023504, 0.00019835382, 0.0, 0.0045495294, 4.594868e-06, 0.00053596497, -0.19740541, -0.00019835394, 2.0, 68.645, 8.0, 1.0000002], [39.85971, 0.010527664, 4.069523e-06, -0.5709858, 1.0023566, 0.00019835662, 0.0, 0.004077424, 4.0696027e-06, -0.0020570308, -0.19740902, -0.00019835673, 2.0, 68.909996, 8.0, 1.0000002], [31.58696, 0.010518163, 3.5871944e-06, -0.5739262, 1.0023571, 0.00019835679, 0.0, 0.0035681943, 3.5872765e-06, -0.0028464794, -0.1974236, -0.00019835692, 2.0, 69.177, 8.0, 1.0000002], [25.104433, 0.010524525, 3.187503e-06, -0.5472355, 1.002358, 0.00019835519, 0.0, 0.0031664027, 3.1875716e-06, 9.62317e-05, -0.19741179, -0.00019835532, 2.0, 69.47, 8.0, 1.0000002], [19.929855, 0.010513833, 2.854198e-06, -0.5067443, 1.0023516, 0.00019835518, 0.0, 0.002815219, 2.8542624e-06, -0.0064308643, -0.1974148, -0.00019835531, 2.0, 69.786, 8.0, 1.0000002], [15.836134, 0.010514904, 2.6090495e-06, -0.44916308, 1.0023596, 0.00019835385, 0.0, 0.0026249092, 2.6091063e-06, -0.0026237965, -0.19741322, -0.00019835398, 2.0, 70.116, 8.0, 1.0000002], [12.600794, 0.010508797, 2.4354974e-06, -0.3855698, 1.0023488, 0.00019834818, 0.0, 0.002462529, 2.435536e-06, 0.0014029741, -0.19740626, -0.0001983483, 2.0, 70.526, 8.0, 1.0000002], [9.990409, 0.0105115315, 2.3121102e-06, -0.32602763, 1.0023568, 0.000198356, 0.0, 0.0023267642, 2.3121531e-06, -0.0027794838, -0.19741975, -0.00019835614, 2.0, 70.94, 8.0, 1.0000002], [7.939562, 0.010514432, 2.223916e-06, -0.26790345, 1.0023516, 0.0001983489, 0.0, 0.0022505752, 2.223943e-06, -0.010918021, -0.19740307, -0.00019834902, 2.0, 71.458, 8.0, 1.0000002], [6.3004045, 0.01050835, 2.1739313e-06, -0.21774375, 1.0023869, 0.00019837428, 0.0, 0.0021737802, 2.1739554e-06, 0.0029451847, -0.19744779, -0.00019837442, 2.0, 72.106, 8.0, 1.0000002], [5.008012, 0.010513099, 2.1390981e-06, -0.17769861, 1.0023885, 0.00019837786, 0.0, 0.0021399907, 2.139111e-06, -0.0033926964, -0.19744599, -0.00019837798, 2.0, 72.918, 8.0, 1.0000002], [3.9859712, 0.010508453, 2.1167896e-06, -0.142865, 1.0023872, 0.0001983794, 0.0, 0.0021188892, 2.1168087e-06, -0.0001296997, -0.19743688, -0.00019837954, 2.0, 73.934, 8.0, 1.0000002], [3.1680837, 0.0105141075, 2.1025605e-06, -0.114314735, 1.0023944, 0.00019838015, 0.0, 0.0021098347, 2.1025867e-06, -0.0030505657, -0.19744438, -0.00019838026, 2.0, 75.209, 8.0, 1.0000002], [2.504006, 0.01051037, 2.088523e-06, -0.09063205, 1.0024015, 0.00019838315, 0.0, 0.0021020023, 2.0885607e-06, 0.00065255165, -0.19744818, -0.00019838328, 2.0, 76.82, 8.0, 1.0000002], [1.9879117, 0.010512401, 2.0865468e-06, -0.072336614, 1.0023866, 0.00019837452, 0.0, 0.002088784, 2.0865878e-06, -0.003677845, -0.19744892, -0.00019837465, 2.0, 78.845, 8.0, 1.0000002], [1.5814751, 0.010510129, 2.0813786e-06, -0.058428645, 1.0023991, 0.00019837692, 0.0, 0.0020913924, 2.081417e-06, -0.0016133785, -0.19745956, -0.00019837705, 2.0, 81.386, 8.0, 1.0000002], [1.2617111, 0.01051464, 2.0801756e-06, -0.045754313, 1.0023983, 0.00019837586, 0.0, 0.0020867614, 2.0802245e-06, 0.0008494854, -0.19745608, -0.00019837597, 2.0, 84.57, 8.0, 1.0000002], [1.0000616, 0.010510105, 2.0764644e-06, -0.03638327, 1.0023925, 0.00019837073, 0.0, 0.002085015, 2.0765144e-06, 0.00040960312, -0.19743952, -0.00019837085, 2.0, 88.582, 8.0, 1.0000002]]
  out "Exit 2":bool=TRUE
  # "Instructions:\nBefore running the VI you must type a valid IP adress that corresponds to the instrument.Then press the Run button to execute this VI.\nWhile this VI is running, choose the available channel, enter the SPEIS parameters or keep the default\n values, then press the start button to begin the experience. \nChoose the waveform to draw : Nyquist, modZ, theta...\nPress the stop button to end experience and the exit button to stop the VI execution."
  # "do N current steps"
  # "from Ei (V)  vs. previous"
  # "to Ef (V) vs. previous"
  # "Before EIS  stay for ts (s)"
  # "and record every dI (A)"
  # "or every dt (s)"
  # "Start EIS from  Fi (Hz)"
  # "sweep linear/logarithmic"
  # "to Ff (Hz)"
  # "for Nf frequencies"
  # "with the amplitude (V)"
  # "wait for Pw"
  # "average Na times"
  # "drift correction"
  # "with I Range"
  # "and bandwidth"
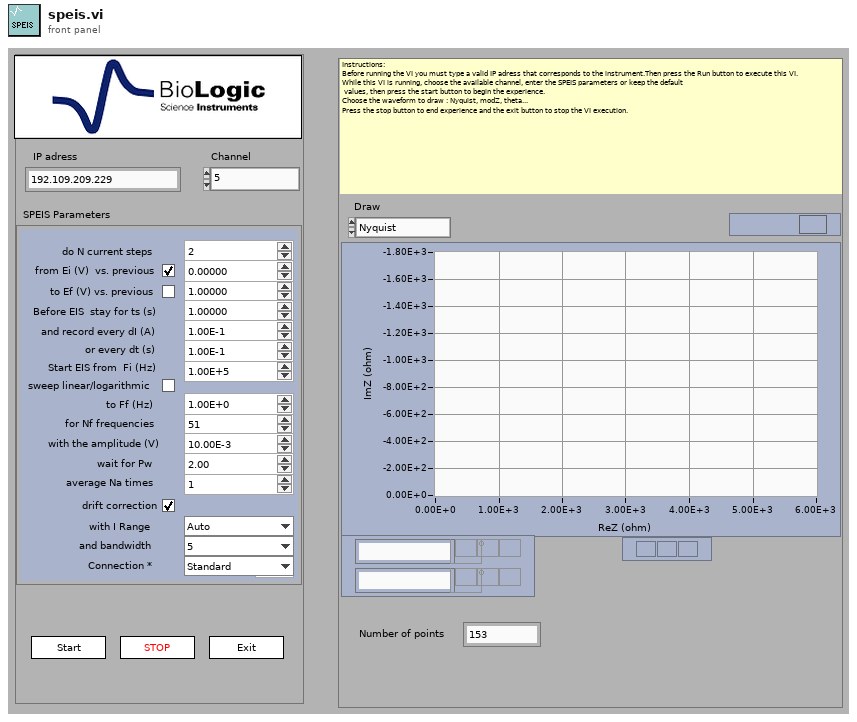
[diagram p1: front panel]
types:
  T1 = enum16{"Nyquist", "modZ", "theta", "modE", "modI", "Edc", "Idc", "E range", "I range", "f(t)"}
  T2 = cluster{"Step_number":i32, "Initial_Voltage_step":sgl, "vs_initial":bool, "Final_Voltage_step":sgl, "vs_final":bool, "Duration_step":sgl, "Record_every_dI":sgl, "Record_every_dT":sgl, "Initial_frequency":sgl, "sweep":bool, "Final_frequency":sgl, "Frequency_number":i32, "Amplitude_Voltage":sgl, "Wait_for_steady":sgl, "Average_N_times":i32, "Correction":bool, "I_Range":u16, "Bandwidth":u16, "em":u16, "ce":u16}
  T3 = typedef "Type Descriptor Enumeration__ogtk.ctl" = enum8{"<Null>", "I8", "I16", "I32", "I64", "U8", "U16", "U32", "U64", "SGL", "DBL", "EXT", "CSG", "CDB", "CXT", "0x0F", "0x10", "0x11", "0x12", "0x13", "0x14", "Enum U8", "Enum U16", "Enum U32", "Enum U64", "SGL PQ", "DBL PQ", "EXT PQ", "CSG PQ", "CDB PQ", "CXT PQ", "0x1F", "0x20", "Boolean", "0x22", "0x23", "0x24", "0x25", "0x26", "0x27", "0x28", "0x29", "0x2A", "0x2B", "0x2C", "0x2D", "0x2E", "0x2F", "String", "0x31", "Path", "Pict", "0x34", "0x35", "0x36", "DAQ", "0x38", "0x39", "0x3A", "0x3B", "0x3C", "0x3D", "0x3E", "0x3F", "Array", "0x41", "0x42", "0x43", "0x44", "0x45", "0x46", "0x47", "0x48", "0x49", "0x4A", "0x4B", "0x4C", "0x4D", "0x4E", "0x4F", "Cluster", "0x51", "0x52", "Variant", "Waveform", "0x55", "0x56", "0x57", "0x58", "0x59", "0x5A", "0x5B", "0x5C", "0x5D", "0x5E", "0x5F", "0x60", "0x61", "0x62", "0x63", "0x64", "0x65", "0x66", "0x67", "0x68", "0x69", "0x6A", "0x6B", "0x6C", "0x6D", "0x6E", "0x6F", "Refnum"}
  T4 = cluster{"Data Type":T3, "Format String":string}[]
  T5 = cluster{"Channel":i32, "BoardVersion":i32, "BoardSerialCode":i32, "FirmwareCode":i32, "FirmwareVersion":i32, "XilinxVersion":i32, "AmpCode":i32, "NbAmp":i32, "LcBoard":i32, "Zboard":i32, "MuxBoard":i32, "GPRAboard":i32, "MemSize":i32, "MemFilled":i32, "state":i32, "MaxIRange":i32, "MinIRange":i32, "MaxBandwidth":i32, "NbOfTechniques":i32}
  T6 = cluster{"Label":string, "type":i32, "valeur":u32, "index":i32}[]
  T7 = cluster{"IRQskipped":i32, "NbRaws":i32, "NbCols":i32, "Technique Index":i32, "TechniqueID":i32, "PrcessIndex":i32, "loop":i32, "StartTime":dbl, "MuxPad":i32}
  T8 = cluster{"State":i32, "MemFilled":i32, "TimeBase":sgl, " Ewe":sgl, " EweRangeMin":sgl, " EweRangeMax":sgl, "Ece":sgl, "EceRangeMin":sgl, "EceRangeMax":sgl, "Eoverflow":i32, "I":sgl, "IRange":i32, "Ioverflow":i32, "ElapsedTime":sgl, "Freq":sgl, "Rcomp":sgl, "Saturation":sgl, "OptErr":i32, "OptPos":i32}
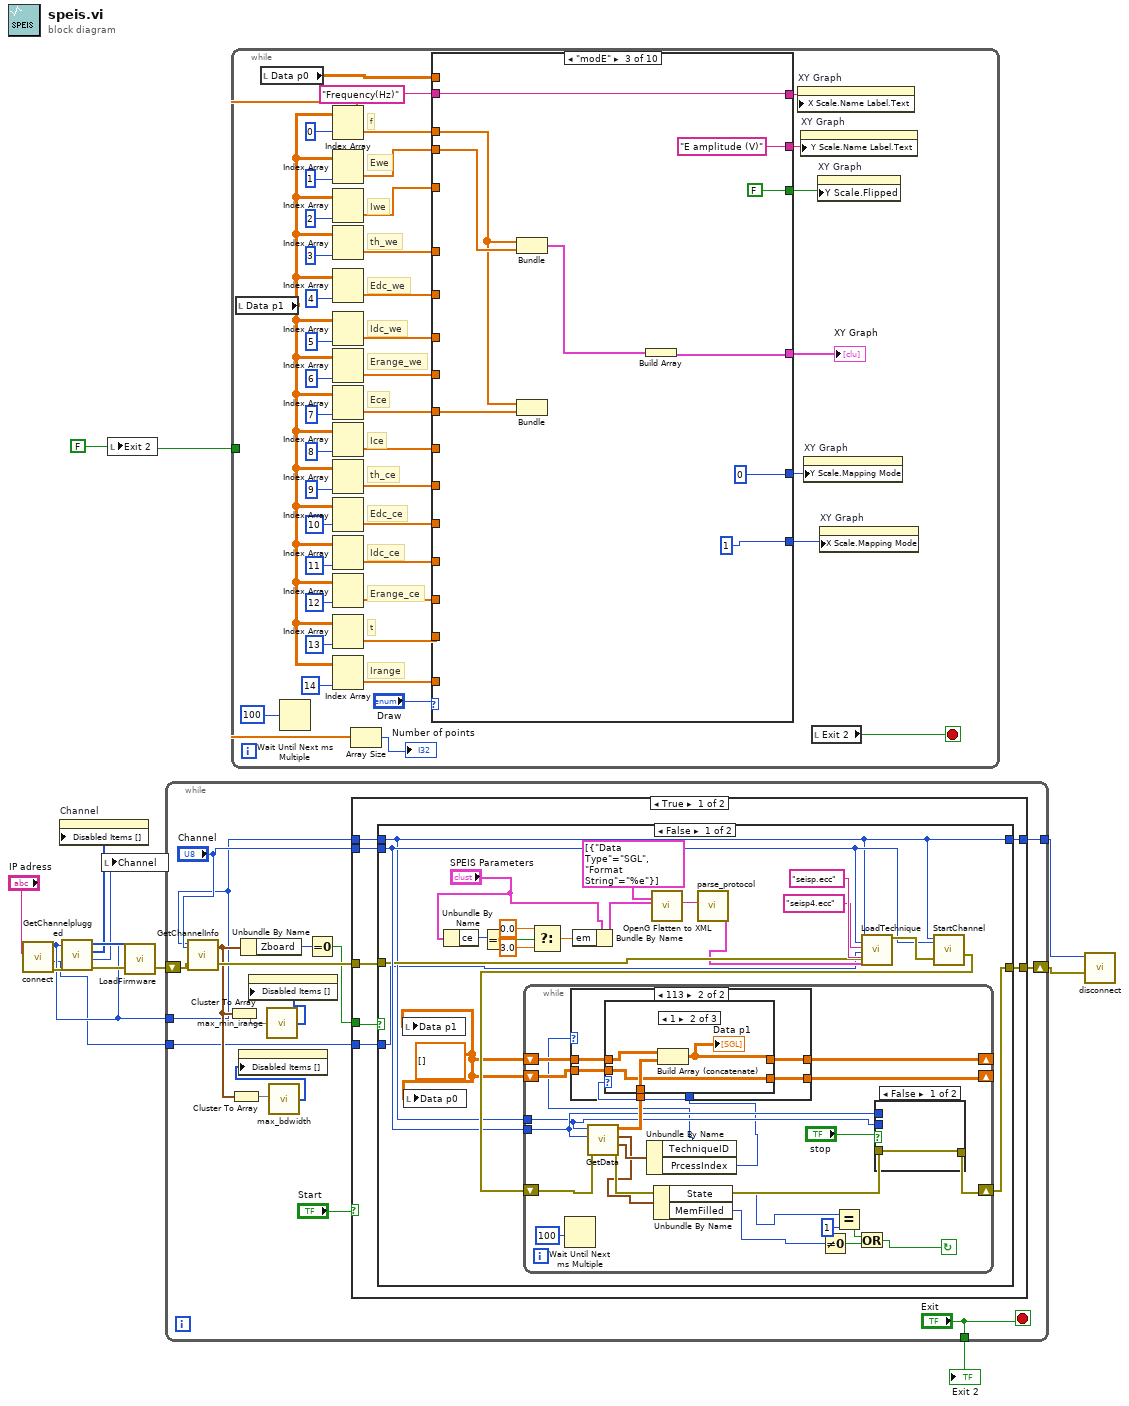
[diagram p0: block diagram]
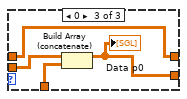
[diagram p4: hidden frame]
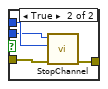
[diagram p5: hidden frame]
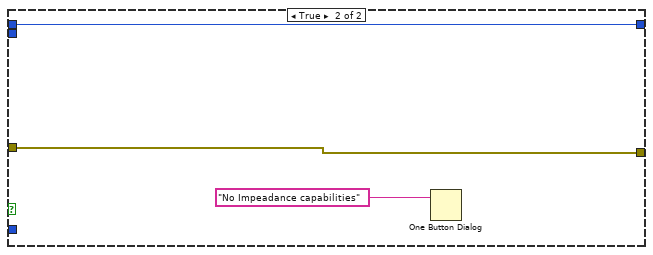
[diagram p6: hidden frame]
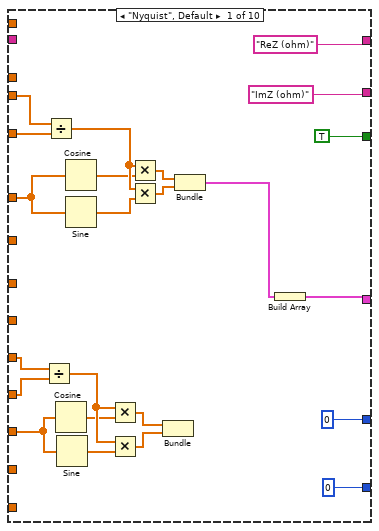
[diagram p8: hidden frame]
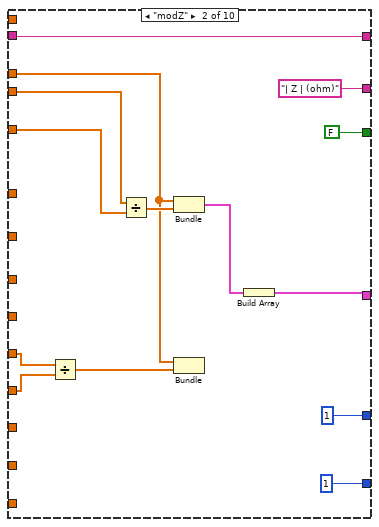
[diagram p9: hidden frame]
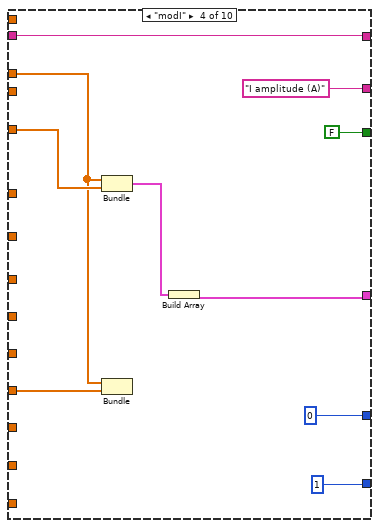
[diagram p10: hidden frame]
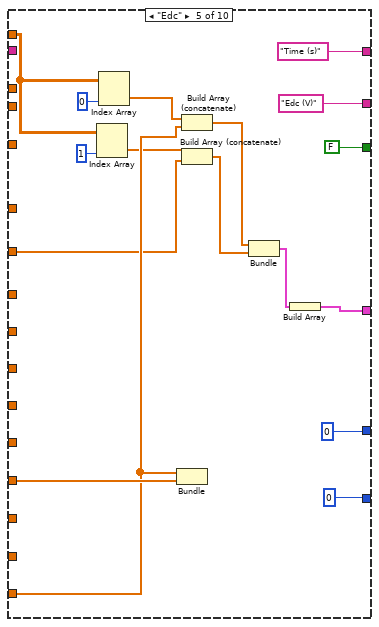
[diagram p11: hidden frame]
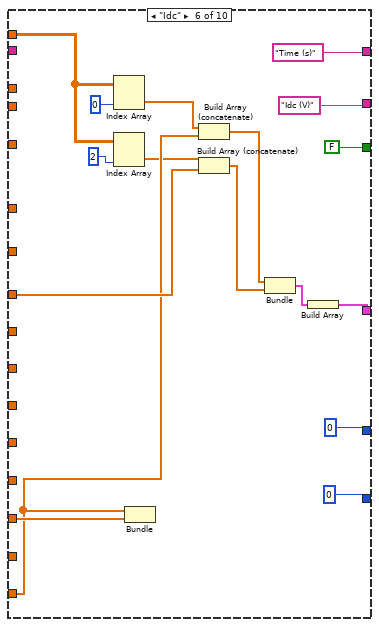
[diagram p12: hidden frame]
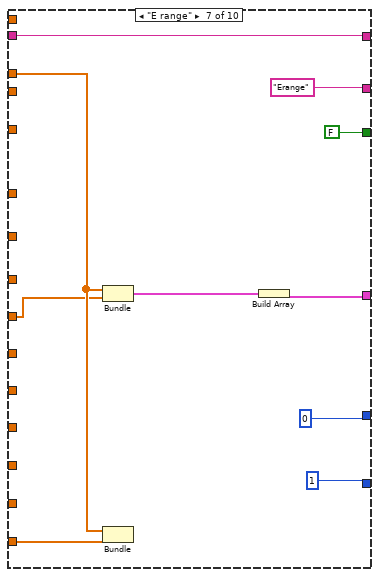
[diagram p13: hidden frame]
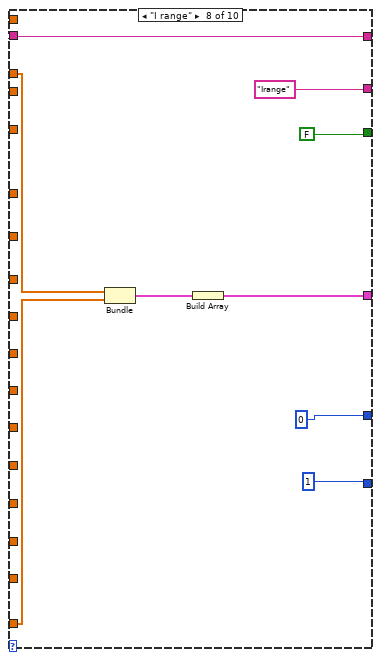
[diagram p14: hidden frame]
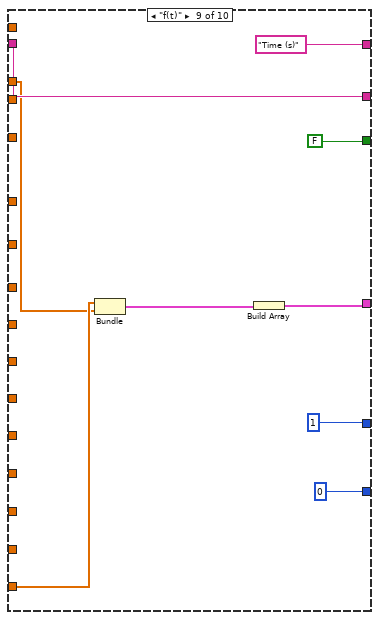
[diagram p15: hidden frame]
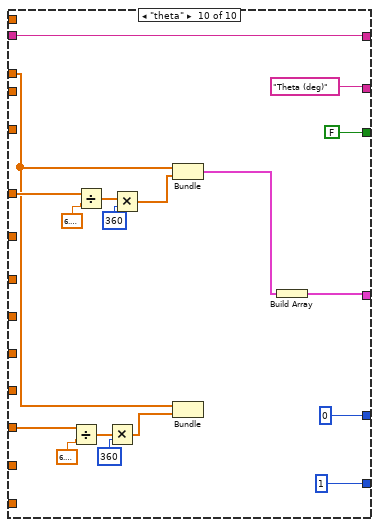
[diagram p16: hidden frame]
diagram:
  w6 = FALSE
  n1 = call "connect.vi"("IP"="IP adress") -> ("error out"=w12:errorcluster, "Device Code"=w1:i32, "ID"=w3:i32)  [unwired: 7 in, 1 out]
  n2 = call "GetChannelplugged.vi"("error in (no error)"=w12, "ID"=w3) -> ("error out"=w10:errorcluster, "First channel"=w8:i32, "Disabled channels"=w7:i32[], "Plugged channels"=w11:i32[])  [unwired: 6 in]
  n3 = property on="Channel" class="Ring (strict)"("Disabled Items []"=w7) -> ()  [unwired: 2 in, 2 out]
  n4 = local write "Channel"(w8) -> ()
  n5 = local write "Exit 2"(w6) -> ()
  n6 = call "LoadFirmware.vi"("error in (no error)"=w10, "Channels"=w11, "ID"=w3) -> ("error out"=w4:errorcluster)  [unwired: 7 in, 1 out]
  n7 = while {
    shift-right: [w28] -> w13
    shift-left: w4 -> [w23]
    tunnel: ["Exit"] -> w5
    tunnel: w3 -> [w16]
    tunnel: [w15] -> w2
    tunnel: w1 -> [w14]
    stop <- "Exit" stop-if-true
    n8 = call "GetChannelInfo.vi"("error in (no error)"=w23, "Channel"="Channel", "ID"=w16) -> ("error out"=w22:errorcluster, "Channel information"=w20:T5)  [unwired: 7 in]
    n9 = Cluster To Array(cluster=w20) -> (array=w26:i32[])
    n10 = Cluster To Array(cluster=w20) -> (array=w19:i32[])
    n11 = Unbundle By Name(w20) -> ("Zboard"=w25:i32)
    n12 = call "max_min_irange.vi"("resources"=w26) -> ("disabled ranges"=w17:i32[])
    n13 = property on="I_Range" class="Ring (strict)"("Disabled Items []"=w17) -> ()  [unwired: 2 in, 2 out]
    n14 = call "max_bdwidth.vi"("resources"=w19) -> ("disabled ranges"=w18:i32[])
    n15 = property on="Bandwidth" class="Ring (strict)"("Disabled Items []"=w18) -> ()  [unwired: 2 in, 2 out]
    n16 = Equal To 0?(x=w25) -> (x = 0?=w21:bool)
    n17 = case shown="True" "Start" {
      tunnel: "Channel" -> [w35 _]
      tunnel: [w36 w106] -> w28
      tunnel: w22 -> [w34 w106]
      tunnel: w21 -> [w33 _]
      tunnel: w16 -> [w32 w105]
      tunnel: [w31 w105] -> w15
      tunnel: w14 -> [w30 _]
      frame True {
        n18 = case shown="False" w33 {
          tunnel: [w53 w103] -> w36
          tunnel: w35 -> [w52 _]
          tunnel: w34 -> [w51 w103]
          tunnel: w32 -> [w46 w102]
          tunnel: [w46 w102] -> w31
          tunnel: w30 -> [w45 _]
          frame False {
            w50 = sgl[][] [] ("Data")
            n19 = local write "Data p1"(w50) -> ()
            n20 = local write "Data p0"(w50) -> ()
            n21 = Unbundle By Name("SPEIS Parameters") -> ("ce"=w40:u16)
            n22 = Equal To 0?(x=w40) -> (x = 0?=w39:bool)
            n23 = Select(t=0.0, s=w39, f=3.0) -> (s? t:f=w43:dbl)
            n24 = Bundle By Name(cluster="SPEIS Parameters", "em"=w43) -> (w37:T2)
            n25 = call "OpenG Flatten to XML.vi"("Type Formats (default)"=T4 [{"Data Type"=enum."SGL", "Format String"="%e"}] ("Type Formats"), "LabVIEW Data"=w37) -> ("XML String"=w49:string)  [unwired: 8 in, 1 out]
            n26 = call "parse_protocol.vi"("XML String In"=w49) -> ("Params Values"=w48:T6)  [unwired: 8 in]
            n27 = call "LoadTechnique.vi"("ID"=w46, "Selected Channel"=w52, "FName4"="seisp4.ecc" ("FName"), "Device Code"=w45, "FName"="seisp.ecc", "Protocol Parameters"=w48, "error in (no error)"=w51) -> ("error out"=w55:errorcluster)  [unwired: 12 in]
            n28 = call "StartChannel.vi"("error in (no error)"=w55, "Channel"=w52, "ID"=w46) -> ("error out"=w54:errorcluster)  [unwired: 8 in]
            n29 = while {
              shift-right: [w73] -> w53
              shift-left: w54 -> [w75]
              tunnel: w52 -> [w64]
              shift-right: [w68] -> _
              shift-left: w50 -> [w69]
              shift-right: [w67] -> _
              shift-left: w50 -> [w66]
              tunnel: w46 -> [w63]
              stop <- w71 continue-if-true
              n30 = Wait Until Next ms Multiple(millisecond multiple=u32 100) -> ()  [unwired: 1 out]
              n31 = call "GetData.vi"("error in (no error)"=w75, "Channel"=w64, "ID"=w63) -> ("error out"=w72:errorcluster, "Data information"=w62:T7, "Current values"=w58:T8, "Data"=w70:dbl[][])  [unwired: 5 in]
              n32 = Unbundle By Name(w62) -> ("TechniqueID"=w61:i32, "PrcessIndex"=w57:i32)
              n33 = case shown="113" w61 {
                tunnel: w70 -> [_ w86]
                tunnel: w69 -> [w80 w85]
                tunnel: [w80 w84] -> w68
                tunnel: [w79 w83] -> w67
                tunnel: w66 -> [w79 w82]
                tunnel: w57 -> [_ w81]
                frame 0, Default {
                }
                frame 113 {
                  n34 = case shown="1" w81 {
                    tunnel: w86 -> [_ w92 w96]
                    tunnel: w85 -> [w88 w91 w93]
                    tunnel: [w88 w90 w93] -> w84
                    tunnel: [w87 w89 w95] -> w83
                    tunnel: w82 -> [w87 w89 w94]
                    frame 2, Default {
                    }
                    frame 1 {
                      n35 = Build Array (concatenate)(w91, w92) -> (w90:dbl[][])
                      "Data p1" <- w90
                    }
                    frame 0 {
                      n36 = Build Array (concatenate)(w94, w96) -> (w95:dbl[][])
                      "Data p0" <- w95
                    }
                  }
                }
              }
              n37 = Unbundle By Name(w58) -> ("State"=w60:i32, "MemFilled"=w59:i32)
              n38 = Not Equal To 0?(x=w59) -> (x != 0?=w76:bool)
              n39 = Equal?(x=w60, y=1) -> (x = y?=w77:bool)
              n40 = Or(x=w77, y=w76) -> (x .or. y?=w71:bool)
              n41 = case shown="False" "stop" {
                tunnel: [w97 w101] -> w73
                tunnel: w72 -> [w97 w100]
                tunnel: w64 -> [_ w99]
                tunnel: w63 -> [_ w98]
                frame False {
                }
                frame True {
                  n42 = call "StopChannel.vi"("error in (no error)"=w100, "Channel"=w99, "ID"=w98) -> ("error out"=w101:errorcluster)  [unwired: 8 in]
                }
              }
            }
          }
          frame True {
            n43 = One Button Dialog(message="No Impeadance capabilities" ("error source (\" \")")) -> ()  [unwired: 1 in, 1 out]
          }
        }
      }
      frame False {
      }
    }
  }
  "Exit 2" <- w5
  n44 = while {
    tunnel: w6 -> [_]
    stop <- w138 stop-if-true
    # "Erange_ce"
    # "Idc_ce"
    # "Edc_ce"
    # "th_ce"
    # "Ice"
    # "Ece"
    # "t"
    # "Irange"
    # "Erange_we"
    # "Idc_we"
    # "Edc_we"
    # "th_we"
    # "Iwe"
    # "Ewe"
    # "f"
    n45 = local read "Data p1"() -> (w123:sgl[][])
    n46 = local read "Data p0"() -> (w110:sgl[][])
    n47 = Wait Until Next ms Multiple(millisecond multiple=u32 100) -> ()  [unwired: 1 out]
    n48 = Index Array(array=w123, index (col)=0 ("Index")) -> (element=w109:sgl[])  [unwired: 1 in]
    n49 = Index Array(array=w123, index (col)=1 ("Index")) -> (element=w124:sgl[])  [unwired: 1 in]
    n50 = Index Array(array=w123, index (col)=2 ("Index")) -> (element=w128:sgl[])  [unwired: 1 in]
    n51 = Index Array(array=w123, index (col)=3 ("Index")) -> (element=w143:sgl[])  [unwired: 1 in]
    n52 = Index Array(array=w123, index (col)=4 ("disabled index (col)")) -> (element=w137:sgl[])  [unwired: 1 in]
    n53 = Index Array(array=w123, index (col)=5 ("disabled index (col)")) -> (element=w134:sgl[])  [unwired: 1 in]
    n54 = Index Array(array=w123, index (col)=6 ("index (row)")) -> (element=w125:sgl[])  [unwired: 1 in]
    n55 = Index Array(array=w123, index (col)=7) -> (element=w116:sgl[])  [unwired: 1 in]
    n56 = Index Array(array=w123, index (col)=8) -> (element=w115:sgl[])  [unwired: 1 in]
    n57 = Index Array(array=w123, index (col)=9) -> (element=w114:sgl[])  [unwired: 1 in]
    n58 = Index Array(array=w123, index (col)=10) -> (element=w113:sgl[])  [unwired: 1 in]
    n59 = Index Array(array=w123, index (col)=11) -> (element=w112:sgl[])  [unwired: 1 in]
    n60 = Index Array(array=w123, index (col)=12) -> (element=w111:sgl[])  [unwired: 1 in]
    n61 = Index Array(array=w123, index (col)=13 ("disabled index (col)")) -> (element=w126:sgl[])  [unwired: 1 in]
    n62 = Index Array(array=w123, index (col)=14 ("disabled index (col)")) -> (element=w127:sgl[])  [unwired: 1 in]
    n63 = Array Size(array=w109) -> (size(s)=→"Number of points":i32)
    n64 = case shown="\"modE\"" "Draw" {
      tunnel: w109 -> [_ w175 w189 w200 _ _ w245 w253 w262 w271]
      tunnel: w124 -> [w172 w186 w196 _ _ _ _ _ _ _]
      tunnel: w128 -> [w171 w179 _ w206 _ _ _ _ _ _]
      tunnel: ["ImZ (ohm)" ("Y Scale.Name Label.Text") "| Z | (ohm)" ("Y Scale.Name Label.Text") "E amplitude (V)" ("Y Scale.Name Label.Text") "I amplitude (A)" ("Y Scale.Name Label.Text") "Edc (V)" ("Y Scale.Name Label.Text") "Idc (V)" ("Y Scale.Name Label.Text") "Erange" ("Y Scale.Name Label.Text") "Irange" ("Y Scale.Name Label.Text") w267 "Theta (deg)" ("Y Scale.Name Label.Text")] -> w145
      tunnel: w143 -> [w170 _ _ _ _ _ _ _ _ w280]
      tunnel: ["ReZ (ohm)" ("Y Scale.Name Label.Text") w183 w194 w204 "Time (s)" ("Y Scale.Name Label.Text") "Time (s)" ("Y Scale.Name Label.Text") w250 w259 "Time (s)" ("Y Scale.Name Label.Text") w286] -> w142
      tunnel: "Frequency(Hz)" ("Y Scale.Name Label.Text") -> [_ w183 w194 w204 _ _ w250 w259 w267 w286]
      tunnel: [TRUE ("Y Scale.Flipped") FALSE ("Y Scale.Flipped") FALSE ("Y Scale.Flipped") FALSE ("Y Scale.Flipped") FALSE ("Y Scale.Flipped") FALSE ("Y Scale.Flipped") FALSE ("Y Scale.Flipped") FALSE FALSE FALSE ("Y Scale.Flipped")] -> w140
      tunnel: [u8 0 ("X Scale.Mapping Mode") u8 1 ("X Scale.Mapping Mode") u8 1 ("X Scale.Mapping Mode") u8 1 ("X Scale.Mapping Mode") 0 0 1 1 0 u8 1 ("X Scale.Mapping Mode")] -> w139
      tunnel: w137 -> [_ _ _ _ w207 _ _ _ _ _]
      tunnel: w134 -> [_ _ _ _ _ w228 _ _ _ _]
      tunnel: w125 -> [_ _ _ _ _ _ w241 _ _ _]
      tunnel: w127 -> [_ _ _ _ _ _ _ w254 _ _]
      tunnel: w126 -> [_ _ _ _ w209 w227 _ _ w263 _]
      tunnel: [0 1 u8 0 ("X Scale.Mapping Mode") u8 0 ("X Scale.Mapping Mode") 0 0 0 0 1 0 ("X Scale.Mapping Mode")] -> w130
      tunnel: w116 -> [w161 w177 w190 _ _ _ _ _ _ _]
      tunnel: w115 -> [w160 w176 _ w199 _ _ _ _ _ _]
      tunnel: w114 -> [w159 _ _ _ _ _ _ _ _ w272]
      tunnel: w113 -> [_ _ _ _ w219 _ _ _ _ _]
      tunnel: w112 -> [_ _ _ _ _ w236 _ _ _ _]
      tunnel: w111 -> [_ _ _ _ _ _ w242 _ _ _]
      tunnel: [w153 w173 w187 w197 w218 w234 w243 w251 w260 w269] -> w107
      tunnel: w110 -> [_ _ _ _ w212 w230 _ _ _ _]
      frame "Nyquist", Default {
        n65 = Divide(x=w161, y=w160) -> (x/y=w155:sgl[])
        n66 = Divide(x=w172, y=w171) -> (x/y=w157:sgl[])
        n67 = Cosine(x=w159) -> (cos(x)=w154:sgl[])
        n68 = Sine(x=w159) -> (sin(x)=w162:sgl[])
        n69 = Cosine(x=w170) -> (cos(x)=w156:sgl[])
        n70 = Sine(x=w170) -> (sin(x)=w152:sgl[])
        n71 = Multiply(x=w155, y=w154) -> (x*y=w164:sgl[])
        n72 = Multiply(x=w155, y=w162) -> (x*y=w163:sgl[])
        n73 = Multiply(x=w157, y=w156) -> (x*y=w151:sgl[])
        n74 = Multiply(x=w157, y=w152) -> (x*y=w150:sgl[])
        n75 = Bundle(w164, w163) -> ()  [unwired: 1 in, 1 out]
        n76 = Bundle(w151, w150) -> (w158:cluster{sgl[], sgl[]})  [unwired: 1 in]
        n77 = Build Array(w158) -> (w153:cluster{sgl[], sgl[]}[])
      }
      frame "modZ" {
        n78 = Divide(x=w177, y=w176) -> (x/y=w178:sgl[])
        n79 = Divide(x=w186, y=w179) -> (x/y=w185:sgl[])
        n80 = Bundle("Data p1"=w175, w185) -> (w174:cluster{"Data p1":sgl[], sgl[]})  [unwired: 1 in]
        n81 = Bundle("Data p1"=w175, w178) -> ()  [unwired: 1 in, 1 out]
        n82 = Build Array(w174) -> (w173:cluster{"Data p1":sgl[], sgl[]}[])
      }
      frame "modE" {
        n83 = Bundle("Data p1"=w189, "Data p1"=w196) -> (w188:cluster{"Data p1":sgl[], "Data p1":sgl[]})  [unwired: 1 in]
        n84 = Bundle("Data p1"=w189, "Data p1"=w190) -> ()  [unwired: 1 in, 1 out]
        n85 = Build Array(w188) -> (w187:cluster{"Data p1":sgl[], "Data p1":sgl[]}[])
      }
      frame "modI" {
        n86 = Bundle("Data p1"=w200, "Data p1"=w206) -> (w198:cluster{"Data p1":sgl[], "Data p1":sgl[]})  [unwired: 1 in]
        n87 = Bundle("Data p1"=w200, "Data p1"=w199) -> ()  [unwired: 1 in, 1 out]
        n88 = Build Array(w198) -> (w197:cluster{"Data p1":sgl[], "Data p1":sgl[]}[])
      }
      frame "Edc" {
        n89 = Index Array(array=w212, index (col)=1 ("Index")) -> (element=w208:sgl[])  [unwired: 1 in]
        n90 = Index Array(array=w212, index (col)=0 ("Index")) -> (element=w210:sgl[])  [unwired: 1 in]
        n91 = Bundle("Data p1"=w209, "Data p1"=w219) -> ()  [unwired: 1 in, 1 out]
        n92 = Build Array (concatenate)(w210, w209) -> (w215:sgl[])
        n93 = Build Array (concatenate)(w208, w207) -> (w214:sgl[])
        n94 = Bundle(w215, w214) -> (w211:cluster{sgl[], sgl[]})  [unwired: 1 in]
        n95 = Build Array(w211) -> (w218:cluster{sgl[], sgl[]}[])
      }
      frame "Idc" {
        n96 = Index Array(array=w230, index (col)=0 ("Index")) -> (element=w229:sgl[])  [unwired: 1 in]
        n97 = Index Array(array=w230, index (col)=2 ("Index")) -> (element=w226:sgl[])  [unwired: 1 in]
        n98 = Bundle("Data p1"=w227, "Data p1"=w236) -> ()  [unwired: 1 in, 1 out]
        n99 = Build Array (concatenate)(w229, w227) -> (w225:sgl[])
        n100 = Build Array (concatenate)(w226, w228) -> (w224:sgl[])
        n101 = Bundle(w225, w224) -> (w235:cluster{sgl[], sgl[]})  [unwired: 1 in]
        n102 = Build Array(w235) -> (w234:cluster{sgl[], sgl[]}[])
      }
      frame "E range" {
        n103 = Bundle("Data p1"=w245, "Data p1"=w241) -> (w244:cluster{"Data p1":sgl[], "Data p1":sgl[]})  [unwired: 1 in]
        n104 = Bundle("Data p1"=w245, "Data p1"=w242) -> ()  [unwired: 1 in, 1 out]
        n105 = Build Array(w244) -> (w243:cluster{"Data p1":sgl[], "Data p1":sgl[]}[])
      }
      frame "I range" {
        n106 = Bundle("Data p1"=w253, "Data p1"=w254) -> (w252:cluster{"Data p1":sgl[], "Data p1":sgl[]})  [unwired: 1 in]
        n107 = Build Array(w252) -> (w251:cluster{"Data p1":sgl[], "Data p1":sgl[]}[])
      }
      frame "f(t)" {
        n108 = Bundle("Data p1"=w263, "Data p1"=w262) -> (w261:cluster{"Data p1":sgl[], "Data p1":sgl[]})  [unwired: 1 in]
        n109 = Build Array(w261) -> (w260:cluster{"Data p1":sgl[], "Data p1":sgl[]}[])
      }
      frame "theta" {
        n110 = Divide(x=w272, y=6.283185307179586) -> (x/y=w274:dbl[])
        n111 = Divide(x=w280, y=6.283185307179586) -> (x/y=w283:dbl[])
        n112 = Multiply(x=w274, y=360) -> (x*y=w276:dbl[])
        n113 = Multiply(x=w283, y=360) -> (x*y=w279:dbl[])
        n114 = Bundle("Data p1"=w271, w279) -> (w270:cluster{"Data p1":sgl[], dbl[]})  [unwired: 1 in]
        n115 = Bundle("Data p1"=w271, w276) -> ()  [unwired: 1 in, 1 out]
        n116 = Build Array(w270) -> (w269:cluster{"Data p1":sgl[], dbl[]}[])
      }
    }
    "XY Graph" <- w107
    n117 = property on="XY Graph" class="XYGraph (strict)"("X Scale.Name Label.Text"=w142) -> ()  [unwired: 2 in, 2 out]
    n118 = property on="XY Graph" class="XYGraph (strict)"("Y Scale.Name Label.Text"=w145) -> ()  [unwired: 2 in, 2 out]
    n119 = property on="XY Graph" class="XYGraph (strict)"("Y Scale.Mapping Mode"=w130) -> ()  [unwired: 2 in, 2 out]
    n120 = local read "Exit 2"() -> (w138:bool)
    n121 = property on="XY Graph" class="XYGraph (strict)"("Y Scale.Flipped"=w140) -> ()  [unwired: 2 in, 2 out]
    n122 = property on="XY Graph" class="XYGraph (strict)"("X Scale.Mapping Mode"=w139) -> ()  [unwired: 2 in, 2 out]
  }
  n123 = call "disconnect.vi"("error in (no error)"=w13, "ID"=w2) -> ()  [unwired: 9 in, 1 out]
